vi "Construct Dictionary.vi"(5 "Dictionary in":refnum<class "Dictionary.lvclass">, 8 "error in (no error)":errorcluster, 11 "Data":cluster{"Key":string, "Value":refnum<class>}[](array[cluster])) -> (0 "error out":errorcluster, 3 "Dictionary":refnum<class "Dictionary.lvclass">)   [LabVIEW 2017, in "Generic Object Serializer Tests.lvlib" / "Dictionary.lvclass"]
uses:
  Dictionary.lvclass
  Dictionary.lvclass/Dictionary.ctl
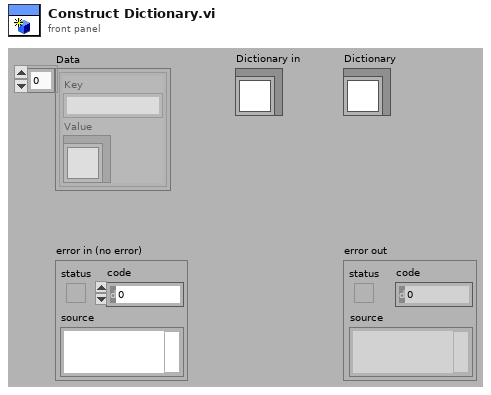
[diagram p1: front panel]
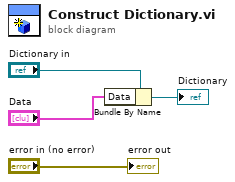
[diagram p0: block diagram]
diagram:
  n1 = Bundle By Name(cluster="Dictionary in", "Data"="Data") -> (→"Dictionary":refnum<class "Dictionary.lvclass">)
  "error out" <- "error in (no error)"
